vi "FTW-CSV-Variant-Traverse.vi"(0 "Variant":variant, 1 "Options":T2={"String Quotes"=FALSE, "Real Format"="%#_15g", "Timestamp Format"="%^<%Y-%m-%dT%H:%M:%S%3uZ>T", "Delimiter"=","}, 5 "Type":T1, 11 "error in":errorcluster) -> (4 "CSV String":string, 15 "error out":errorcluster)   [LabVIEW 2015]
uses:
  FTW-CSV-SerializeOptions.ctl
  <vilib>/Utility/Data Type/Type Definitions/Data Type.ctl
  <vilib>/Utility/Data Type/NI_Data Type.lvlib
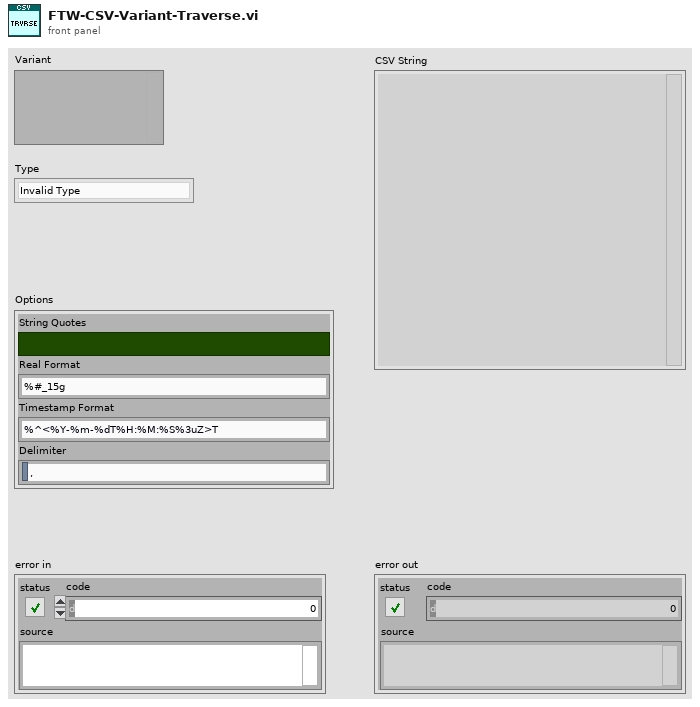
[diagram p1: front panel]
types:
  T1 = typedef "NI_Data Type.lvlib/Data Type.ctl" = enum8{"Invalid Type", "Void", "I8", "I16", "I32", "I64", "U8", "U16", "U32", "U64", "Single Float", "Double Float", "Extended Float", "Single Complex", "Double Complex", "Extended Complex", "Enum U8", "Enum U16", "Enum U32", "Enum U64", "Single Float With Unit", "Double Float With Unit", "Extended Float With Unit", "Single Complex with Unit", "Double Complex with Unit", "Extended Complex with Unit", "Boolean", "String", "Path", "Picture", "Tag", "Array", "Cluster", "Variant", "LV Variant", "Waveform", "Timestamp", "Digital Waveform", "Digital Data", "ExpressData", "Refnum", "External Data", "VI", "Poly VI", "LabVIEW Class Instance", "Fixed Point"}
  T2 = typedef "FTW-CSV-SerializeOptions.ctl" = cluster{"String Quotes":bool, "Real Format":string, "Timestamp Format":string, "Delimiter":string}
  T3 = typedef "NI_Data Type.lvlib/Refnum Type.ctl" = enum16{"NotARefnum", "UnknownRefnum", "Generic", "Datalog", "ByteStream", "Device", "Occurence", "TCPNetConnection", "Auto", "Menu", "Imaq", "Hardware", "DataSocket", "Visa", "IVI", "UDPNetConnection", "Notifier", "Queue", "Irda", "EventReg", "DotNet", "UserEvent", "Callback", "UNUSED_EMPTY_POSITION", "BlueToothNetConnection", "LVObjApp", "LVObjVI", "LVObjUnknown", "GenericClass", "UserDefinedRefnumTag", "DataValue", "RT FIFO", "TDMS File"}
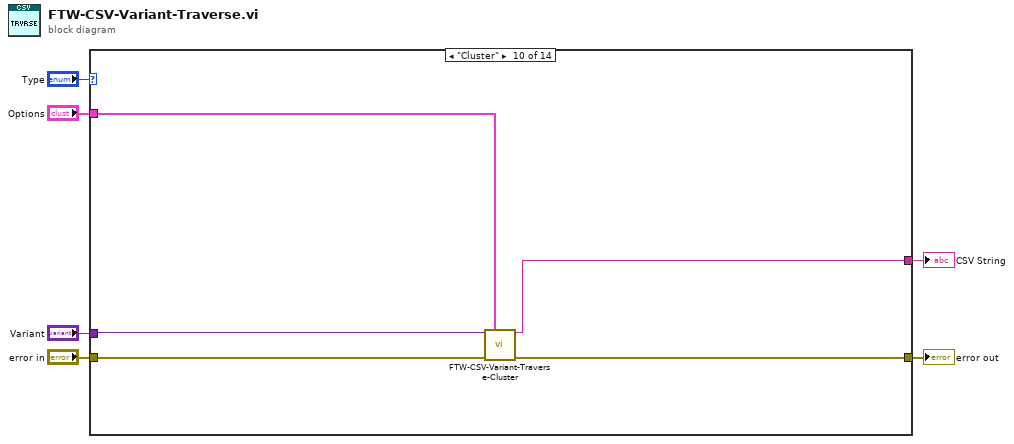
[diagram p0: block diagram]
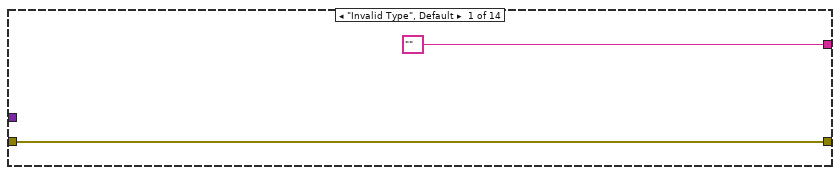
[diagram p2: hidden frame]
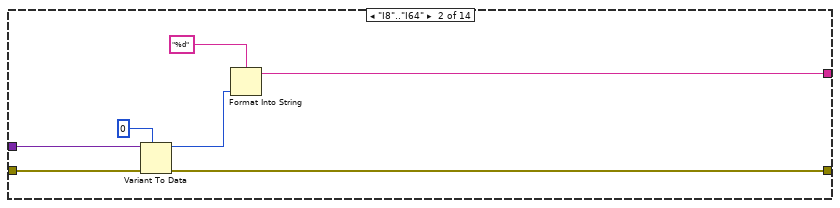
[diagram p3: hidden frame]
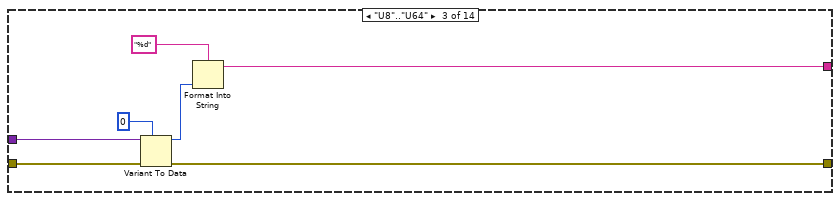
[diagram p4: hidden frame]
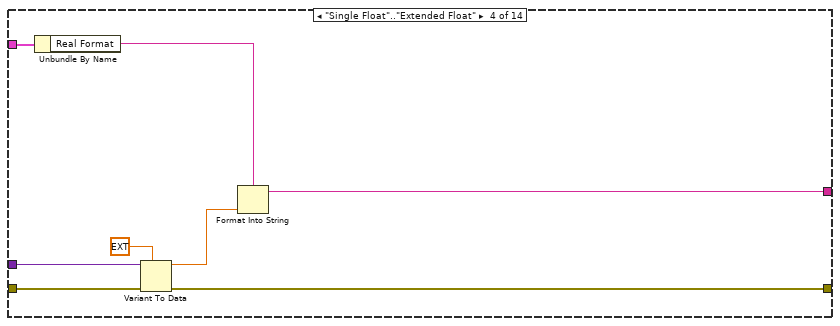
[diagram p5: hidden frame]
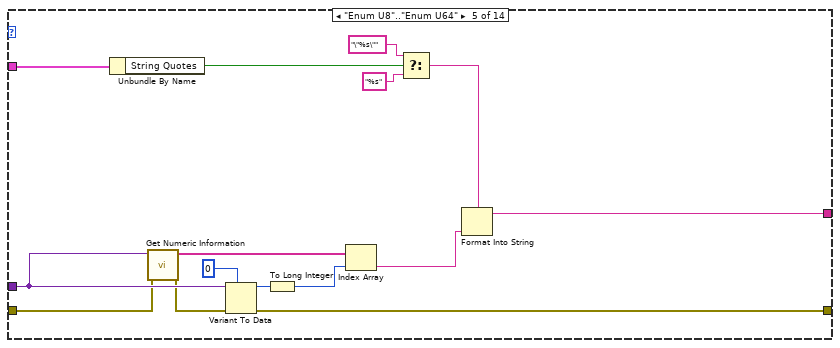
[diagram p6: hidden frame]
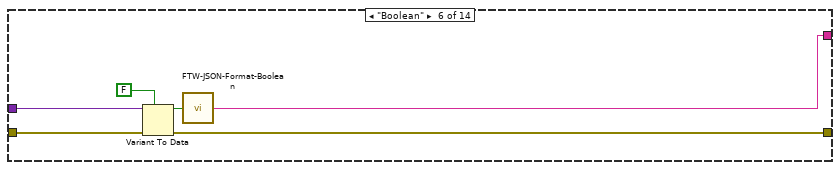
[diagram p7: hidden frame]
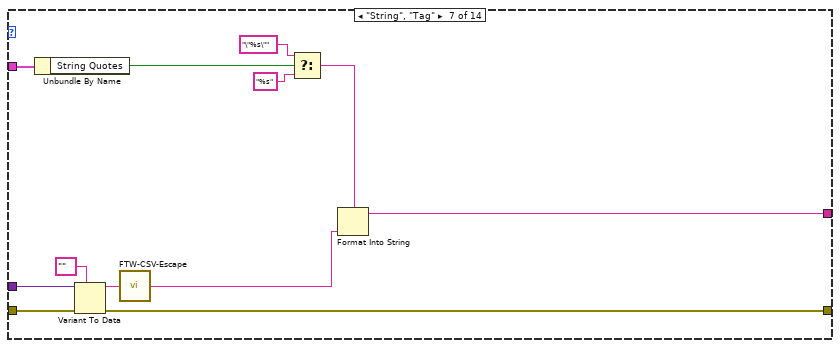
[diagram p8: hidden frame]
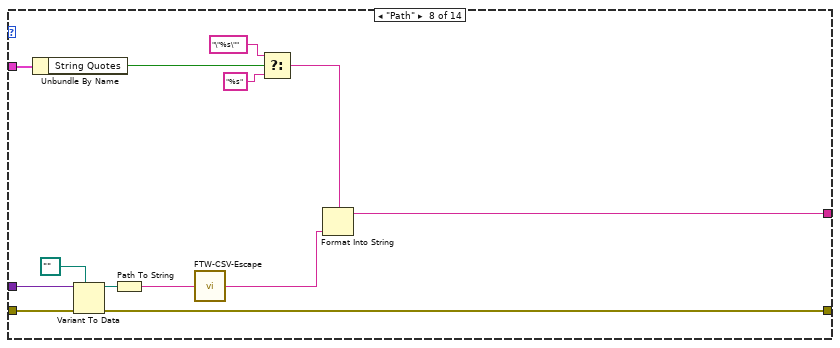
[diagram p9: hidden frame]
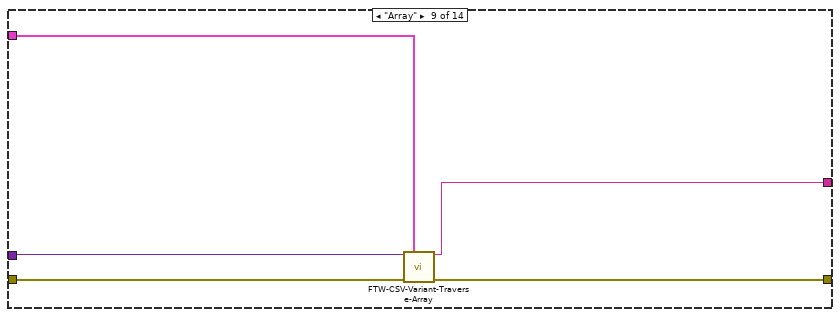
[diagram p10: hidden frame]
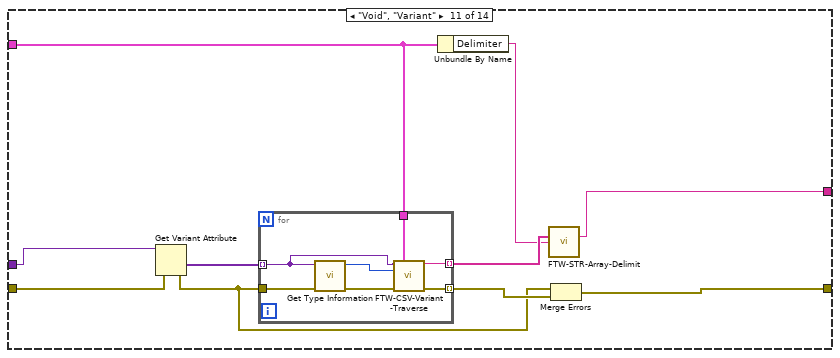
[diagram p11: hidden frame]
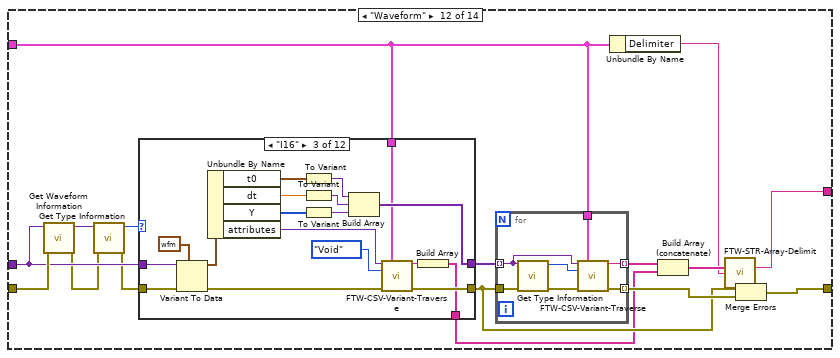
[diagram p12: hidden frame]
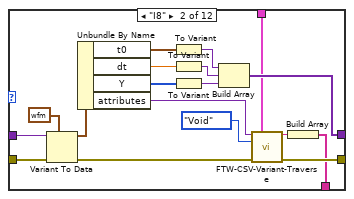
[diagram p14: hidden frame]
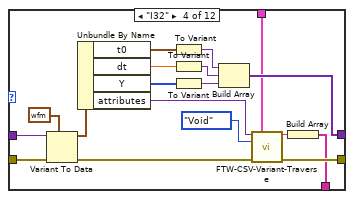
[diagram p15: hidden frame]
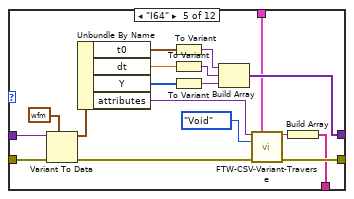
[diagram p16: hidden frame]
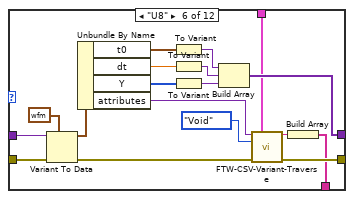
[diagram p17: hidden frame]
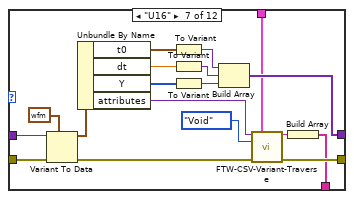
[diagram p18: hidden frame]
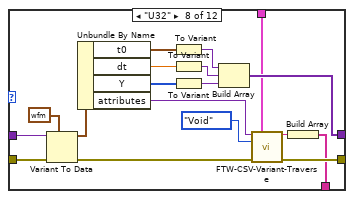
[diagram p19: hidden frame]
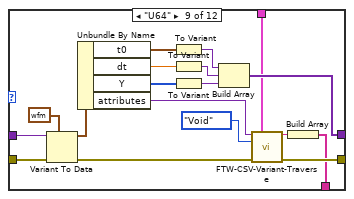
[diagram p20: hidden frame]
diagram:
  n1 = case shown="\"Cluster\"" "Type" {
    tunnel: "error in" -> [w8 w15 w22 w30 w37 w51 w63 w76 w81 w86 w96 w119 w333 w343]
    tunnel: [w8 w14 w21 w29 w45 w50 w62 w75 w80 w85 w92 w115 w332 w345] -> w5
    tunnel: ["" ("empty string") w11 w18 w27 w44 w47 w60 w73 w77 w82 w93 w116 w330 w344] -> w4
    tunnel: "Variant" -> [_ w13 w20 w28 w38 w49 w61 w74 w79 w84 w91 w113 w331 w341]
    tunnel: "Options" -> [_ _ _ w24 w35 _ w53 w65 w78 w83 w88 w105 w328 w335]
    frame "Invalid Type", Default {
    }
    frame "I8".."I64" {
      n2 = Variant To Data(error in=w15, type=i64 0, Variant=w13) -> (data=w10:i64, error out=w14:errorcluster)
      n3 = Format Into String(format string="%d", w10) -> (resulting string=w11:string)  [unwired: 2 in, 1 out]
    }
    frame "U8".."U64" {
      n4 = Variant To Data(error in=w22, type=u64 0, Variant=w20) -> (data=w17:u64, error out=w21:errorcluster)
      n5 = Format Into String(format string="%d", w17) -> (resulting string=w18:string)  [unwired: 2 in, 1 out]
    }
    frame "Single Float".."Extended Float" {
      n6 = Unbundle By Name(w24) -> ("Real Format"=w23:string)
      n7 = Variant To Data(error in=w30, type=ext 0.0, Variant=w28) -> (data=w26:ext, error out=w29:errorcluster)
      n8 = Format Into String(format string=w23, w26) -> (resulting string=w27:string)  [unwired: 2 in, 1 out]
    }
    frame "Enum U8".."Enum U64" {
      n9 = Unbundle By Name(w35) -> ("String Quotes"=w34:bool)
      n10 = call <vilib>:"Get Numeric Information.vi"("error in (no error)"=w37, "Variant"=w38) -> ("error out"=w36:errorcluster, "Enum Names"=w42:string[])  [unwired: 6 in, 2 out]
      n11 = Variant To Data(error in=w36, type=u64 0, Variant=w38) -> (data=w41:u64, error out=w45:errorcluster)
      n12 = To Long Integer(number=w41) -> (32bit integer=w40:i32)
      n13 = Index Array(array=w42, index=w40) -> (element=w39:string)
      n14 = Select(t="\"%s\"" ("format string"), s=w34, f="%s" ("format string")) -> (s? t:f=w32:string)
      n15 = Format Into String(format string=w32, w39) -> (resulting string=w44:string)  [unwired: 2 in, 1 out]
    }
    frame "Boolean" {
      n16 = Variant To Data(error in=w51, type=FALSE, Variant=w49) -> (data=w46:bool, error out=w50:errorcluster)
      n17 = call "FTW-JSON-Format-Boolean.vi"("LabVIEW Boolean"=w46) -> ("JSON Boolean"=w47:string)
    }
    frame "String", "Tag" {
      n18 = Unbundle By Name(w53) -> ("String Quotes"=w56:bool)
      n19 = Variant To Data(error in=w63, type="" ("empty string"), Variant=w61) -> (data=w59:string, error out=w62:errorcluster)
      n20 = call "FTW-CSV-Escape.vi"("String"=w59) -> ("Escaped UTF-8 String"=w57:string)
      n21 = Select(t="\"%s\"" ("format string"), s=w56, f="%s" ("format string")) -> (s? t:f=w52:string)
      n22 = Format Into String(format string=w52, w57) -> (resulting string=w60:string)  [unwired: 2 in, 1 out]
    }
    frame "Path" {
      n23 = Unbundle By Name(w65) -> ("String Quotes"=w68:bool)
      n24 = Variant To Data(error in=w76, type=path "", Variant=w74) -> (data=w72:path, error out=w75:errorcluster)
      n25 = Path To String(path=w72) -> (string=w69:string)
      n26 = call "FTW-CSV-Escape.vi"("String"=w69) -> ("Escaped UTF-8 String"=w71:string)
      n27 = Select(t="\"%s\"" ("format string"), s=w68, f="%s" ("format string")) -> (s? t:f=w64:string)
      n28 = Format Into String(format string=w64, w71) -> (resulting string=w73:string)  [unwired: 2 in, 1 out]
    }
    frame "Array" {
      n29 = call "FTW-CSV-Variant-Traverse-Array.vi"("Variant"=w79, "Options"=w78, "error in"=w81) -> ("CSV String"=w77:string, "error out"=w80:errorcluster)  [unwired: 11 in]
    }
    frame "Cluster" {
      n30 = call "FTW-CSV-Variant-Traverse-Cluster.vi"("Variant"=w84, "Options"=w83, "error in"=w86) -> ("CSV String"=w82:string, "error out"=w85:errorcluster)  [unwired: 11 in]
    }
    frame "Void", "Variant" {
      n31 = Get Variant Attribute(Variant=w91, error in=w96) -> (values=w89:variant[], error out=w90:errorcluster)  [unwired: 2 in, 2 out]
      n32 = for {
        tunnel: w89 -> [w98] mode=indexing
        tunnel: [w102] -> w94 mode=indexing
        tunnel: w90 -> [w100]
        tunnel: [w103] -> w95 mode=indexing
        tunnel: w88 -> [w101]
        n33 = call <vilib>:"Get Type Information.vi"("error in (no error)"=w100, "Variant"=w98) -> ("error out"=w99:errorcluster, "Type"=w97:T1)  [unwired: 5 in, 3 out]
        n34 = call "FTW-CSV-Variant-Traverse.vi"("Variant"=w98, "Options"=w101, "Type"=w97, "error in"=w99) -> ("CSV String"=w102:string, "error out"=w103:errorcluster)  [unwired: 10 in]
      }
      n35 = Unbundle By Name(w88) -> ("Delimiter"=w87:string)
      n36 = call "FTW-STR-Array-Delimit.vi"("Array of Strings"=w94, "Delimiter"=w87) -> ("Delimited String"=w93:string)  [unwired: 13 in]
      n37 = Merge Errors(w90, w95) -> (w92:errorcluster)
    }
    frame "Waveform" {
      n38 = call <vilib>:"Get Waveform Information.vi"("error in (no error)"=w119, "Variant"=w113) -> ("error out"=w110:errorcluster, "Y Array Type"=w111:variant)  [unwired: 8 in]
      n39 = call <vilib>:"Get Type Information.vi"("error in (no error)"=w110, "Variant"=w111) -> ("error out"=w109:errorcluster, "Type"=w108:T1)  [unwired: 5 in, 3 out]
      n40 = case shown="\"I16\"" w108 {
        tunnel: [w120 w126 w144 w162 w180 w198 w216 w234 w252 w270 w288 w306] -> w114
        tunnel: w113 -> [_ w130 w148 w166 w184 w202 w220 w238 w256 w274 w292 w310]
        tunnel: [_ w138 w156 w174 w192 w210 w228 w246 w264 w282 w300 w318] -> w112
        tunnel: w109 -> [w120 w134 w152 w170 w188 w206 w224 w242 w260 w278 w296 w314]
        tunnel: w105 -> [_ w125 w143 w161 w179 w197 w215 w233 w251 w269 w287 w305]
        tunnel: [_ w121 w139 w157 w175 w193 w211 w229 w247 w265 w283 w301] -> w106
        frame "Invalid Type", Default {
        }
        frame "I8" {
          n41 = Variant To Data(error in=w134, type=waveform(i8) {"t0"=timestamp(0 s since 1904-01-01), "dt"=1.0, "Y"=[]} ("Waveform"), Variant=w130) -> (data=w128:waveform(i8), error out=w127:errorcluster)
          n42 = Unbundle By Name(w128) -> ("t0"=w133:timestamp, "dt"=w132:dbl, "Y"=w131:i8[], "attributes"=w124:variant)
          n43 = To Variant(anything=w133) -> (Variant=w137:variant)
          n44 = To Variant(anything=w132) -> (Variant=w136:variant)
          n45 = To Variant(anything=w131) -> (Variant=w135:variant)
          n46 = Build Array(w137, w136, w135) -> (w138:variant[])
          n47 = call "FTW-CSV-Variant-Traverse.vi"("Variant"=w124, "Options"=w125, "Type"=Data_Type."Void", "error in"=w127) -> ("CSV String"=w122:string, "error out"=w126:errorcluster)  [unwired: 10 in]
          n48 = Build Array(w122) -> (w121:string[])
        }
        frame "I16" {
          n49 = Variant To Data(error in=w152, type=waveform(i16) {"t0"=timestamp(0 s since 1904-01-01), "dt"=1.0, "Y"=[]} ("Waveform"), Variant=w148) -> (data=w146:waveform(i16), error out=w145:errorcluster)
          n50 = Unbundle By Name(w146) -> ("t0"=w151:timestamp, "dt"=w150:dbl, "Y"=w149:i16[], "attributes"=w142:variant)
          n51 = To Variant(anything=w151) -> (Variant=w155:variant)
          n52 = To Variant(anything=w150) -> (Variant=w154:variant)
          n53 = To Variant(anything=w149) -> (Variant=w153:variant)
          n54 = Build Array(w155, w154, w153) -> (w156:variant[])
          n55 = call "FTW-CSV-Variant-Traverse.vi"("Variant"=w142, "Options"=w143, "Type"=Data_Type."Void", "error in"=w145) -> ("CSV String"=w140:string, "error out"=w144:errorcluster)  [unwired: 10 in]
          n56 = Build Array(w140) -> (w139:string[])
        }
        frame "I32" {
          n57 = Variant To Data(error in=w170, type=waveform(i32) {"t0"=timestamp(0 s since 1904-01-01), "dt"=1.0, "Y"=[]} ("Waveform"), Variant=w166) -> (data=w164:waveform(i32), error out=w163:errorcluster)
          n58 = Unbundle By Name(w164) -> ("t0"=w169:timestamp, "dt"=w168:dbl, "Y"=w167:i32[], "attributes"=w160:variant)
          n59 = To Variant(anything=w169) -> (Variant=w173:variant)
          n60 = To Variant(anything=w168) -> (Variant=w172:variant)
          n61 = To Variant(anything=w167) -> (Variant=w171:variant)
          n62 = Build Array(w173, w172, w171) -> (w174:variant[])
          n63 = call "FTW-CSV-Variant-Traverse.vi"("Variant"=w160, "Options"=w161, "Type"=Data_Type."Void", "error in"=w163) -> ("CSV String"=w158:string, "error out"=w162:errorcluster)  [unwired: 10 in]
          n64 = Build Array(w158) -> (w157:string[])
        }
        frame "I64" {
          n65 = Variant To Data(error in=w188, type=waveform(i64) {"t0"=timestamp(0 s since 1904-01-01), "dt"=1.0, "Y"=[]} ("Waveform"), Variant=w184) -> (data=w182:waveform(i64), error out=w181:errorcluster)
          n66 = Unbundle By Name(w182) -> ("t0"=w187:timestamp, "dt"=w186:dbl, "Y"=w185:i64[], "attributes"=w178:variant)
          n67 = To Variant(anything=w187) -> (Variant=w191:variant)
          n68 = To Variant(anything=w186) -> (Variant=w190:variant)
          n69 = To Variant(anything=w185) -> (Variant=w189:variant)
          n70 = Build Array(w191, w190, w189) -> (w192:variant[])
          n71 = call "FTW-CSV-Variant-Traverse.vi"("Variant"=w178, "Options"=w179, "Type"=Data_Type."Void", "error in"=w181) -> ("CSV String"=w176:string, "error out"=w180:errorcluster)  [unwired: 10 in]
          n72 = Build Array(w176) -> (w175:string[])
        }
        frame "U8" {
          n73 = Variant To Data(error in=w206, type=waveform(u8) {"t0"=timestamp(0 s since 1904-01-01), "dt"=1.0, "Y"=[]} ("Waveform"), Variant=w202) -> (data=w200:waveform(u8), error out=w199:errorcluster)
          n74 = Unbundle By Name(w200) -> ("t0"=w205:timestamp, "dt"=w204:dbl, "Y"=w203:u8[], "attributes"=w196:variant)
          n75 = To Variant(anything=w205) -> (Variant=w209:variant)
          n76 = To Variant(anything=w204) -> (Variant=w208:variant)
          n77 = To Variant(anything=w203) -> (Variant=w207:variant)
          n78 = Build Array(w209, w208, w207) -> (w210:variant[])
          n79 = call "FTW-CSV-Variant-Traverse.vi"("Variant"=w196, "Options"=w197, "Type"=Data_Type."Void", "error in"=w199) -> ("CSV String"=w194:string, "error out"=w198:errorcluster)  [unwired: 10 in]
          n80 = Build Array(w194) -> (w193:string[])
        }
        frame "U16" {
          n81 = Variant To Data(error in=w224, type=waveform(u16) {"t0"=timestamp(0 s since 1904-01-01), "dt"=1.0, "Y"=[]} ("Waveform"), Variant=w220) -> (data=w218:waveform(u16), error out=w217:errorcluster)
          n82 = Unbundle By Name(w218) -> ("t0"=w223:timestamp, "dt"=w222:dbl, "Y"=w221:u16[], "attributes"=w214:variant)
          n83 = To Variant(anything=w223) -> (Variant=w227:variant)
          n84 = To Variant(anything=w222) -> (Variant=w226:variant)
          n85 = To Variant(anything=w221) -> (Variant=w225:variant)
          n86 = Build Array(w227, w226, w225) -> (w228:variant[])
          n87 = call "FTW-CSV-Variant-Traverse.vi"("Variant"=w214, "Options"=w215, "Type"=Data_Type."Void", "error in"=w217) -> ("CSV String"=w212:string, "error out"=w216:errorcluster)  [unwired: 10 in]
          n88 = Build Array(w212) -> (w211:string[])
        }
        frame "U32" {
          n89 = Variant To Data(error in=w242, type=waveform(u32) {"t0"=timestamp(0 s since 1904-01-01), "dt"=1.0, "Y"=[]} ("Waveform"), Variant=w238) -> (data=w236:waveform(u32), error out=w235:errorcluster)
          n90 = Unbundle By Name(w236) -> ("t0"=w241:timestamp, "dt"=w240:dbl, "Y"=w239:u32[], "attributes"=w232:variant)
          n91 = To Variant(anything=w241) -> (Variant=w245:variant)
          n92 = To Variant(anything=w240) -> (Variant=w244:variant)
          n93 = To Variant(anything=w239) -> (Variant=w243:variant)
          n94 = Build Array(w245, w244, w243) -> (w246:variant[])
          n95 = call "FTW-CSV-Variant-Traverse.vi"("Variant"=w232, "Options"=w233, "Type"=Data_Type."Void", "error in"=w235) -> ("CSV String"=w230:string, "error out"=w234:errorcluster)  [unwired: 10 in]
          n96 = Build Array(w230) -> (w229:string[])
        }
        frame "U64" {
          n97 = Variant To Data(error in=w260, type=waveform(u64) {"t0"=timestamp(0 s since 1904-01-01), "dt"=1.0, "Y"=[]} ("Waveform"), Variant=w256) -> (data=w254:waveform(u64), error out=w253:errorcluster)
          n98 = Unbundle By Name(w254) -> ("t0"=w259:timestamp, "dt"=w258:dbl, "Y"=w257:u64[], "attributes"=w250:variant)
          n99 = To Variant(anything=w259) -> (Variant=w263:variant)
          n100 = To Variant(anything=w258) -> (Variant=w262:variant)
          n101 = To Variant(anything=w257) -> (Variant=w261:variant)
          n102 = Build Array(w263, w262, w261) -> (w264:variant[])
          n103 = call "FTW-CSV-Variant-Traverse.vi"("Variant"=w250, "Options"=w251, "Type"=Data_Type."Void", "error in"=w253) -> ("CSV String"=w248:string, "error out"=w252:errorcluster)  [unwired: 10 in]
          n104 = Build Array(w248) -> (w247:string[])
        }
        frame "Single Float" {
          n105 = Variant To Data(error in=w278, type=waveform(sgl) {"t0"=timestamp(0 s since 1904-01-01), "dt"=1.0, "Y"=[]} ("Waveform"), Variant=w274) -> (data=w272:waveform(sgl), error out=w271:errorcluster)
          n106 = Unbundle By Name(w272) -> ("t0"=w277:timestamp, "dt"=w276:dbl, "Y"=w275:sgl[], "attributes"=w268:variant)
          n107 = To Variant(anything=w277) -> (Variant=w281:variant)
          n108 = To Variant(anything=w276) -> (Variant=w280:variant)
          n109 = To Variant(anything=w275) -> (Variant=w279:variant)
          n110 = Build Array(w281, w280, w279) -> (w282:variant[])
          n111 = call "FTW-CSV-Variant-Traverse.vi"("Variant"=w268, "Options"=w269, "Type"=Data_Type."Void", "error in"=w271) -> ("CSV String"=w266:string, "error out"=w270:errorcluster)  [unwired: 10 in]
          n112 = Build Array(w266) -> (w265:string[])
        }
        frame "Double Float" {
          n113 = Variant To Data(error in=w296, type=waveform(dbl) {"t0"=timestamp(0 s since 1904-01-01), "dt"=1.0, "Y"=[]} ("Waveform"), Variant=w292) -> (data=w290:waveform(dbl), error out=w289:errorcluster)
          n114 = Unbundle By Name(w290) -> ("t0"=w295:timestamp, "dt"=w294:dbl, "Y"=w293:dbl[], "attributes"=w286:variant)
          n115 = To Variant(anything=w295) -> (Variant=w299:variant)
          n116 = To Variant(anything=w294) -> (Variant=w298:variant)
          n117 = To Variant(anything=w293) -> (Variant=w297:variant)
          n118 = Build Array(w299, w298, w297) -> (w300:variant[])
          n119 = call "FTW-CSV-Variant-Traverse.vi"("Variant"=w286, "Options"=w287, "Type"=Data_Type."Void", "error in"=w289) -> ("CSV String"=w284:string, "error out"=w288:errorcluster)  [unwired: 10 in]
          n120 = Build Array(w284) -> (w283:string[])
        }
        frame "Extended Float" {
          n121 = Variant To Data(error in=w314, type=waveform(ext) {"t0"=timestamp(0 s since 1904-01-01), "dt"=1.0, "Y"=[]} ("Waveform"), Variant=w310) -> (data=w308:waveform(ext), error out=w307:errorcluster)
          n122 = Unbundle By Name(w308) -> ("t0"=w313:timestamp, "dt"=w312:dbl, "Y"=w311:ext[], "attributes"=w304:variant)
          n123 = To Variant(anything=w313) -> (Variant=w317:variant)
          n124 = To Variant(anything=w312) -> (Variant=w316:variant)
          n125 = To Variant(anything=w311) -> (Variant=w315:variant)
          n126 = Build Array(w317, w316, w315) -> (w318:variant[])
          n127 = call "FTW-CSV-Variant-Traverse.vi"("Variant"=w304, "Options"=w305, "Type"=Data_Type."Void", "error in"=w307) -> ("CSV String"=w302:string, "error out"=w306:errorcluster)  [unwired: 10 in]
          n128 = Build Array(w302) -> (w301:string[])
        }
      }
      n129 = for {
        tunnel: w112 -> [w320] mode=indexing
        tunnel: [w323] -> w117 mode=indexing
        tunnel: w114 -> [w325]
        tunnel: [w324] -> w118 mode=indexing
        tunnel: w105 -> [w322]
        n130 = call <vilib>:"Get Type Information.vi"("error in (no error)"=w325, "Variant"=w320) -> ("error out"=w321:errorcluster, "Type"=w319:T1)  [unwired: 5 in, 3 out]
        n131 = call "FTW-CSV-Variant-Traverse.vi"("Variant"=w320, "Options"=w322, "Type"=w319, "error in"=w321) -> ("CSV String"=w323:string, "error out"=w324:errorcluster)  [unwired: 10 in]
      }
      n132 = Unbundle By Name(w105) -> ("Delimiter"=w104:string)
      n133 = Build Array (concatenate)(w117, w106) -> (w107:string[])
      n134 = call "FTW-STR-Array-Delimit.vi"("Array of Strings"=w107, "Delimiter"=w104) -> ("Delimited String"=w116:string)  [unwired: 13 in]
      n135 = Merge Errors(w114, w118) -> (w115:errorcluster)
    }
    frame "Timestamp" {
      n136 = Unbundle By Name(w328) -> ("Timestamp Format"=w326:string)
      n137 = Variant To Data(error in=w333, type=timestamp(0 s since 1904-01-01), Variant=w331) -> (data=w327:timestamp, error out=w332:errorcluster)
      n138 = Format Into String(format string=w326, w327) -> (resulting string=w330:string)  [unwired: 2 in, 1 out]
    }
    frame "Refnum" {
      n139 = Unbundle By Name(w335) -> ("String Quotes"=w338:bool)
      n140 = call <vilib>:"Get Refnum Information.vi"("error in (no error)"=w343, "Variant"=w341) -> ("error out"=w342:errorcluster, "Strict Type"=w339:variant, "Reference Type"=w340:T3)  [unwired: 6 in, 1 out]
      n141 = Select(t="\"%s\"" ("format string"), s=w338, f="%s" ("format string")) -> (s? t:f=w334:string)
      n142 = case shown="\"ByteStream\"..\"TCPNetConnection\", \"UDPNetConnection\"..\"Queue\", \"EventReg\"..\"UserEvent\", \"LVObjApp\"..\"LVObjUnknown\", \"DataValue\"..\"TDMS File\"" w340 {
        tunnel: [w347 w350 w362] -> w345
        tunnel: ["" ("empty string") w353 w361] -> w344
        tunnel: w342 -> [w347 w350 w357]
        tunnel: w341 -> [_ w349 w356]
        tunnel: w339 -> [_ _ _]
        tunnel: w334 -> [_ _ w355]
        frame "NotARefnum", Default {
        }
        frame "ByteStream".."TCPNetConnection", "UDPNetConnection".."Queue", "EventReg".."UserEvent", "LVObjApp".."LVObjUnknown", "DataValue".."TDMS File" {
          n143 = Variant To Flattened String(Variant=w349) -> (data string=w348:string)  [unwired: 1 out]
          n144 = Type Cast(type=u32 0 ("empty string"), x=w348) -> (*(type *) &x=w351:u32)
          n145 = Format Into String(format string="%d", w351) -> (resulting string=w353:string)  [unwired: 2 in, 1 out]
        }
        frame "Visa", "UserDefinedRefnumTag" {
          n146 = Variant To Data(error in=w357, type="" ("empty string"), Variant=w356) -> (data=w360:string, error out=w362:errorcluster)
          n147 = call "FTW-CSV-Escape.vi"("String"=w360) -> ("Escaped UTF-8 String"=w358:string)
          n148 = Format Into String(format string=w355, w358) -> (resulting string=w361:string)  [unwired: 2 in, 1 out]
        }
      }
    }
  }
  "error out" <- w5
  "CSV String" <- w4
